vi "Filtering.vi"(0 "Right border":sgl, 1 "width":u32=5, 3 "height":u32=5, 5 "Left border":sgl, 9 "Bottom border":sgl, 11 "fps":sgl, 12 "F_x":dbl, 13 "F_y":dbl, 14 "h":dbl) -> (4 "distance":sgl, 6 "lateral distance":sgl, 10 "relative speed":sgl)   [LabVIEW 2020]
uses:
  <vilib>/ptbypt/NI_PtbyPt.lvlib
panel:
  out "Distance graph":dbl(graph)
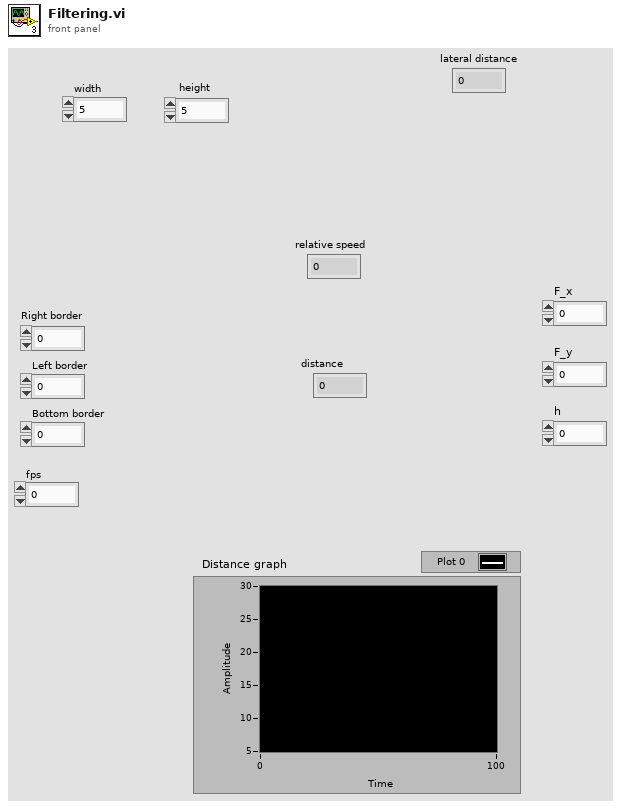
[diagram p1: front panel]
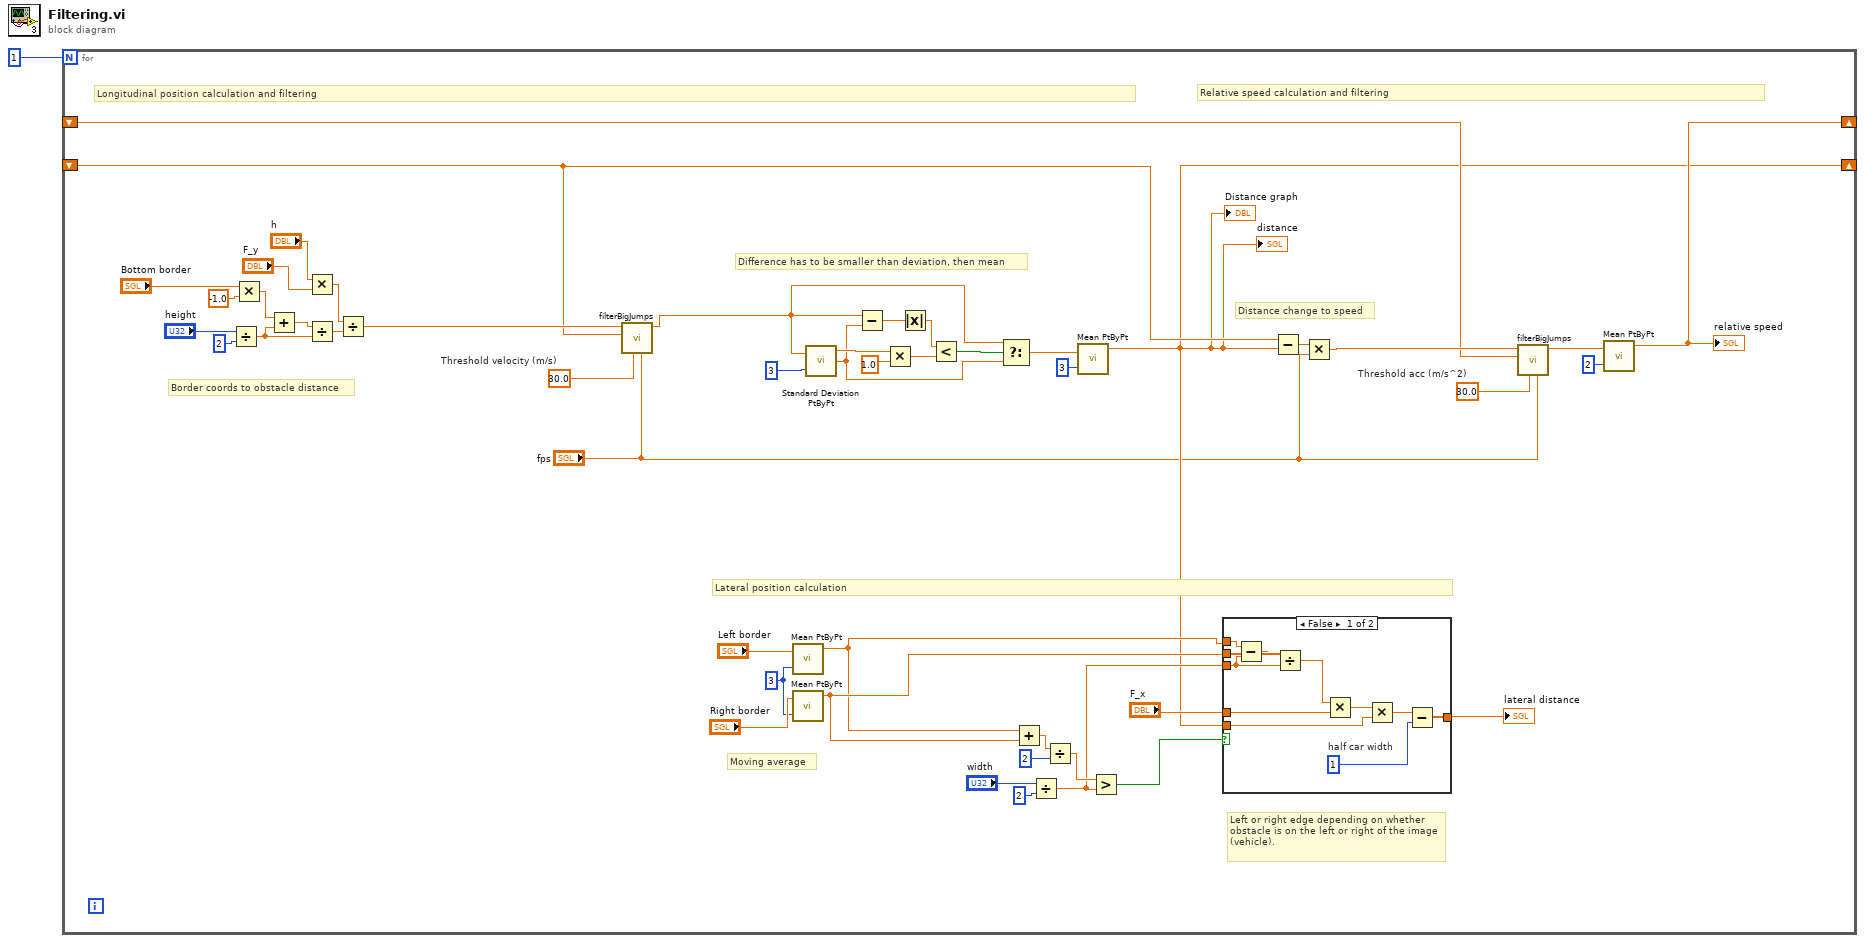
[diagram p0: block diagram]
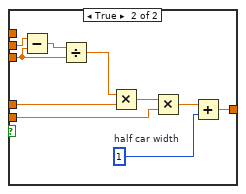
[diagram p2: hidden frame]
diagram:
  n1 = for {
    N: 1 -> [_]
    shift-right: [w3] -> _
    shift-left: _ -> [w9]
    shift-right: [w12] -> _
    shift-left: _ -> [w7]
    w6 = 30.0  # Threshold acc (m/s^2)
    w11 = 30.0  # Threshold velocity (m/s)
    w18 = 3 ("sample length")
    # "Relative speed calculation and filtering"
    # "Longitudinal position calculation and filtering"
    # "Distance change to speed"
    # "Difference has to be smaller than deviation, then mean"
    # "Border coords to obstacle distance"
    # "Left or right edge depending on whether obstacle is on the left or right of the image (vehicle)."
    # "Moving average"
    # "Lateral position calculation"
    n2 = Divide(x="height", y=2) -> (x/y=w36:dbl)
    n3 = Multiply(x="Bottom border", y=sgl -1.0) -> (x*y=w35:sgl)
    n4 = Add(x=w35, y=w36) -> (x+y=w47:dbl)
    n5 = Multiply(x="h", y="F_y") -> (x*y=w49:dbl)
    n6 = Divide(x=w47, y=w36) -> (x/y=w48:dbl)
    n7 = Divide(x=w49, y=w48) -> (x/y=w10:dbl)
    n8 = call "filterBigJumps.vi"("FPS"="fps", "threshold value"=w11, "prev final value"=w9, "calc value"=w10) -> ("filtered value"=w4:dbl)  [unwired: 7 in]
    n9 = call <vilib>:"Mean PtByPt.vi"("x"="Left border", "sample length"=w18) -> ("mean"=w30:dbl)  [unwired: 2 in, 1 out]
    n10 = call <vilib>:"Mean PtByPt.vi"("x"="Right border", "sample length"=w18) -> ("mean"=w31:dbl)  [unwired: 2 in, 1 out]
    n11 = call <vilib>:"Standard Deviation PtByPt.vi"("x"=w4, "sample length"=3) -> ("standard deviation"=w26:dbl, "mean"=w19:dbl)  [unwired: 1 in, 1 out]
    n12 = Subtract(x=w4, y=w19) -> (x-y=w25:dbl)
    n13 = Multiply(x=w26, y=1.0) -> (x*y=w22:dbl)
    n14 = Absolute Value(x=w25) -> (abs(x)=w24:dbl)
    n15 = Less?(x=w24, y=w22) -> (x < y?=w23:bool)
    n16 = Select(t=w4, s=w23, f=w19) -> (s? t:f=w21:dbl)
    n17 = Add(x=w30, y=w31) -> (x+y=w46:dbl)
    n18 = Divide(x="width", y=2) -> (x/y=w39:dbl)
    n19 = Divide(x=w46, y=2) -> (x/y=w44:dbl)
    n20 = call <vilib>:"Mean PtByPt.vi"("x"=w21, "sample length"=3) -> ("mean"=w3:dbl)  [unwired: 2 in, 1 out]
    "distance" <- w3
    "Distance graph" <- w3
    n21 = Greater?(x=w44, y=w39) -> (0:w43:bool)
    n22 = case shown="False" w43 {
      tunnel: w31 -> [_ w69]
      tunnel: w39 -> [w52 w67]
      tunnel: w3 -> [w53 w64]
      tunnel: [w54 w61] -> w42
      tunnel: w30 -> [w51 _]
      tunnel: "F_x" -> [w50 w60]
      frame False {
        w55 = 1  # half car width
        n23 = Subtract(x=w51, y=w52) -> (x-y=w56:dbl)
        n24 = Divide(x=w56, y=w52) -> (x/y=w57:dbl)
        n25 = Multiply(x=w57, y=w50) -> (x*y=w58:dbl)
        n26 = Multiply(x=w58, y=w53) -> (x*y=w59:dbl)
        n27 = Subtract(x=w59, y=w55) -> (x-y=w54:dbl)
      }
      frame True {
        w63 = 1  # half car width
        n28 = Subtract(x=w69, y=w67) -> (x-y=w68:dbl)
        n29 = Divide(x=w68, y=w67) -> (x/y=w66:dbl)
        n30 = Multiply(x=w66, y=w60) -> (x*y=w65:dbl)
        n31 = Multiply(x=w65, y=w64) -> (x*y=w62:dbl)
        n32 = Add(x=w62, y=w63) -> (x+y=w61:dbl)
      }
    }
    "lateral distance" <- w42
    n33 = Subtract(x=w9, y=w3) -> (x-y=w17:dbl)
    n34 = Multiply(x=w17, y="fps") -> (x*y=w8:dbl)
    n35 = call "filterBigJumps.vi"("FPS"="fps", "threshold value"=w6, "prev final value"=w7, "calc value"=w8) -> ("filtered value"=w5:dbl)  [unwired: 7 in]
    n36 = call <vilib>:"Mean PtByPt.vi"("x"=w5, "sample length"=2) -> ("mean"=w12:dbl)  [unwired: 2 in, 1 out]
    "relative speed" <- w12
  }
